vi "Init_UCI.vi"(8 "error in (no error)":errorcluster) -> (0 "error out":errorcluster, 3 "Number of Devices":i32)   [LabVIEW 2010, in "FEMTO_LUCI-10.lvlib"]
doc: "This function enumerates all available LUCI-10 devices."
uses:
  <userlib>/FEMTO/FEMTO_LUCI-10.lvlib
  <userlib>/FEMTO/LUCI_10.dll
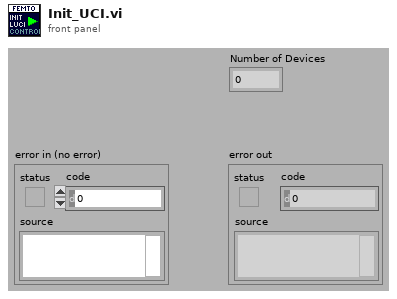
[diagram p1: front panel]
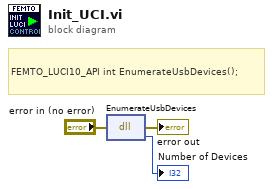
[diagram p0: block diagram]
diagram:
  # "FEMTO_LUCI10_API int EnumerateUsbDevices();"
  n1 = dll-call lib="C:/Program Files (x86)/National Instruments/LabVIEW 2010/user.lib/FEMTO/LUCI_10.dll" fn="EnumerateUsbDevices"(error in="error in (no error)") -> (error out=→"error out":errorcluster, "return type"=→"Number of Devices":i32)  [unwired: 2 in, 1 out]
